vi "Shoot.vi"   [LabVIEW 2019]
uses:
  Robot Global Data.vi
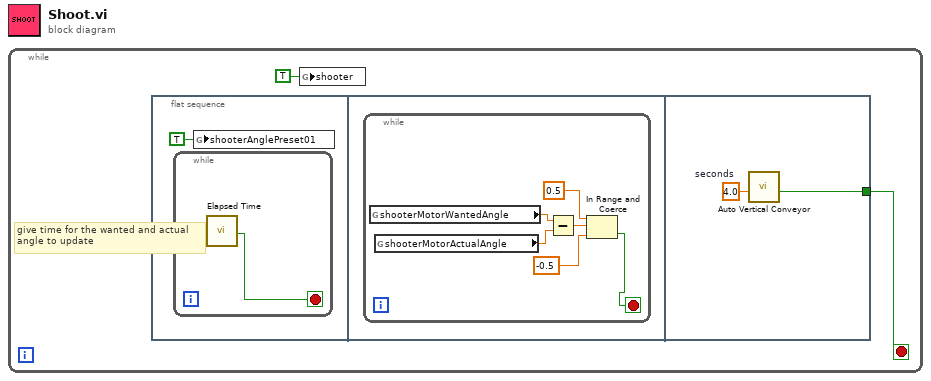
[diagram p0: block diagram]
diagram:
  n1 = while {
    stop <- w1 stop-if-true
    # "give time for the wanted and actual\nangle to update"
    n2 = flat-sequence {
      tunnel: [w11] -> w1
      frame #0 {
        n3 = while {
          stop <- w4 stop-if-true
          n4 = call "Elapsed Time"() -> ("Time has Elapsed"=w4:bool)  [unwired: 12 in, 7 out]
        }
        n5 = global write "Robot Global Data.vi" "shooterAnglePreset01"(TRUE ("shooterAnglePreset01")) -> ()
      }
      frame #1 {
        n6 = while {
          stop <- w10 stop-if-true
          n7 = global read "Robot Global Data.vi" "shooterMotorWantedAngle"() -> (w8:dbl)
          n8 = global read "Robot Global Data.vi" "shooterMotorActualAngle"() -> (w7:dbl)
          n9 = Subtract(x=w8, y=w7) -> (x-y=w9:dbl)
          n10 = In Range and Coerce(upper limit=0.5, x=w9, lower limit=-0.5) -> (In Range?=w10:bool)  [unwired: 1 out]
        }
      }
      frame #2 {
        w12 = 4.0  # seconds
        n11 = call "Auto Vertical Conveyor.vi"("seconds"=w12) -> ("stop"=w11:bool)  [unwired: 10 in]
      }
    }
    n12 = global write "Robot Global Data.vi" "shooter"(TRUE ("shooter")) -> ()
  }
